vi "GlobalRefnum.vi"() -> ()   [LabVIEW 2019]
panel:
  in  "shooter2":string
  in  "shooter1":string
  in  "rightStick":string
  in  "rightBack":string
  in  "rightFront":string
  in  "leftBack":string
  in  "leftStick":string="leftStick"
  in  "leftFront":string="leftFront"
  # "Drive Motors-Refnums"
  # "Joystick Refnums"
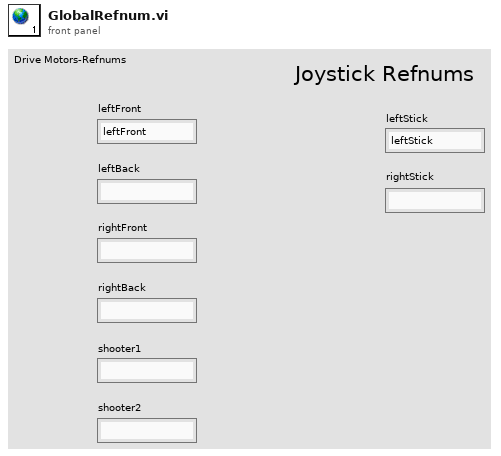
[diagram p1: front panel]
diagram:
